vi "act-20-Initialisation conditionné.vi"() -> ()   [LabVIEW 2010]
uses:
  act/lv_07/lv_07.lvlib
panel:
  out "Ccpc nv":dbl
  out "T init":dbl
  in  "Ccpc anc":dbl
  in  "Cc":dbl
  in  "T":dbl
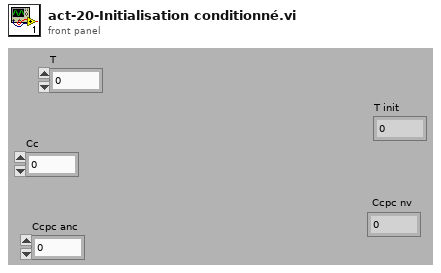
[diagram p1: front panel]
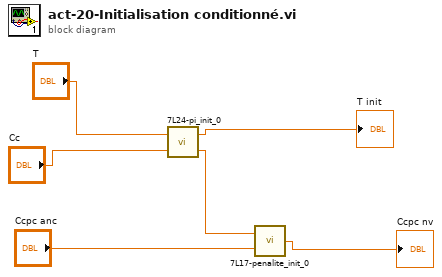
[diagram p0: block diagram]
diagram:
  n1 = call "7L24-pi_init_0.vi"("Cc"="Cc", "T"="T") -> ("Cc init"=w3:dbl, "T init"=→"T init":dbl)
  n2 = call "7L17-penalite_init_0.vi"("Ccpc"="Ccpc anc", "Cc"=w3) -> ("Ccpc init"=→"Ccpc nv":dbl)
